vi "Configure Multiple Instrument Behavior.vi"(7 "Auto Ranging Mode (0: Single Instrument)":u16(ring) items=["Single Instrument", "Multiple Instrument"], 8 "error in (no error)":errorcluster, 10 "Soak Time (0 s)":dbl format="%.2g", 11 "VISA resource name":refnum<visa-resource-name>) -> (0 "error out":errorcluster, 3 "VISA resource name out":refnum<visa-resource-name>)   [LabVIEW 2018, in "Keithley 24XX.lvlib"]
doc: "Configures the time spent by the instrument autoranging during the first acquisition in a sweep. This is especially useful if using a multiple source setup."
uses:
  Keithley 24XX.lvlib
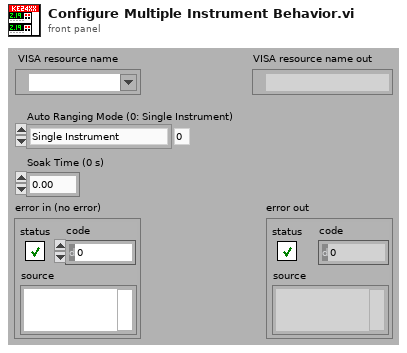
[diagram p1: front panel]
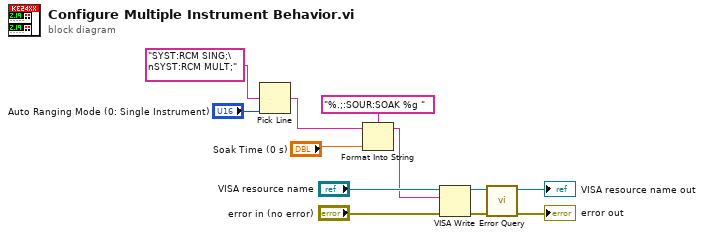
[diagram p0: block diagram]
diagram:
  n1 = Pick Line(multi-line string="SYST:RCM SING;\nSYST:RCM MULT;", line index="Auto Ranging Mode (0: Single Instrument)") -> (output string=w1:string)  [unwired: 1 in]
  n2 = Format Into String(format string="%.;:SOUR:SOAK %g ", initial string=w1, "Soak Time (0 s)") -> (resulting string=w4:string)  [unwired: 1 in, 1 out]
  n3 = VISA Write(VISA resource name="VISA resource name", write buffer=w4, error in (no error)="error in (no error)") -> (VISA resource name out=w8:refnum<visa-resource-name>, error out=w7:errorcluster)  [unwired: 1 out]
  n4 = call "Error Query.vi"("error in (no error)"=w7, "VISA resource name"=w8) -> ("error out"=→"error out":errorcluster, "VISA resource name out"=→"VISA resource name out":refnum<visa-resource-name>)  [unwired: 6 in, 2 out]
